vi "updateNots.vi"(8 "error in (no error)":errorcluster, 11 "reference in":refnum<class "Notification Controller.lvclass">) -> (0 "error out":errorcluster, 3 "reference out":refnum<class "Notification Controller.lvclass">)   [LabVIEW 2014, in "Notification Controller.lvclass"]
uses:
  Notification Controller.lvclass
  Devices Controller_llb/deviceType.ctl
  Devices Controller_llb/Devices Controller.lvclass
  APP/itemsNotification_class/itemsNotification.lvclass
  APP/trackingNotification_class/trackingNotification.lvclass
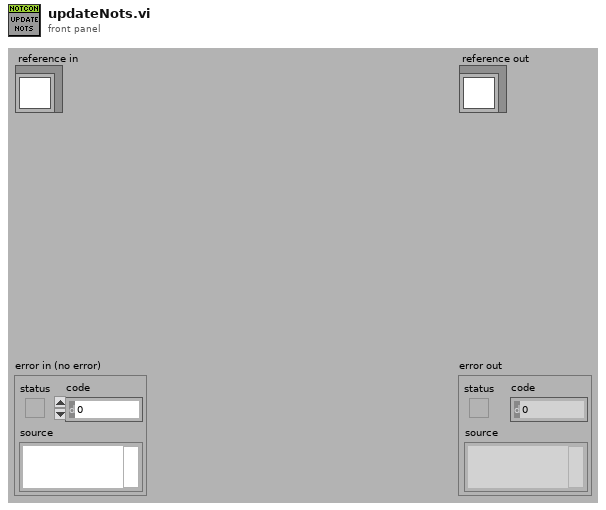
[diagram p1: front panel]
types:
  T1 = typedef "Devices Controller.lvclass/deviceType.ctl" = enum16{"k5", "k4b2", "fitmate", "cpet", "rmr", "bodyBoxPft", "bp", "pp"}
  T2 = cluster{"deviceType":T1, "S/N":string, "SW":string, "Description":string, "Account":string, "System's Location":string, "End User":string, "Email":string, "City":string, "LastChange":string, "Service By":string, "Exp Date":string, "FollowUp Sent":string, "FollowUp Accepted":string, "Note":string}
  T3 = typedef "Notification Controller.lvclass/ObjectAttributesRef.ctl" = refnum<data-value>
  T4 = typedef "Notification Controller.lvclass/ObjectAttributes.ctl" = cluster{"MyAttribute":dbl, "items_data":string[][][], "items_notification_refs":refnum<class "itemsNotification.lvclass">[], "notifications_data_items":string[][], "items_nots?":bool, "devices_controller_ref":refnum<class "Devices Controller.lvclass">, "onlineUpdate":timestamp, "notController?":bool, "tracking_notification_ref":refnum<class "trackingNotification.lvclass">, "notifications_data_tracking":string[][], "tracking_parts_data":string[][], "tracking_nots?":bool, "index_tracking_not":i32[], "file_controller_ref":refnum<class "File Controller.lvclass">}
  T5 = cluster{"notifications_data_items[0]":string, "notifications_data_items[1]":string, "notifications_data_items[2]":string, "notifications_data_items[3]":string, "notifications_data_items[4]":string, "notifications_data_items[5]":string, "notifications_data_items[6]":string, "notifications_data_items[7]":string, "notifications_data_items[8]":string}
  T6 = cluster{"[0]":string, "[1]":string, "[2]":string, "[3]":string, "[4]":string, "[5]":string, "[6]":string, "[7]":string, "[8]":string}
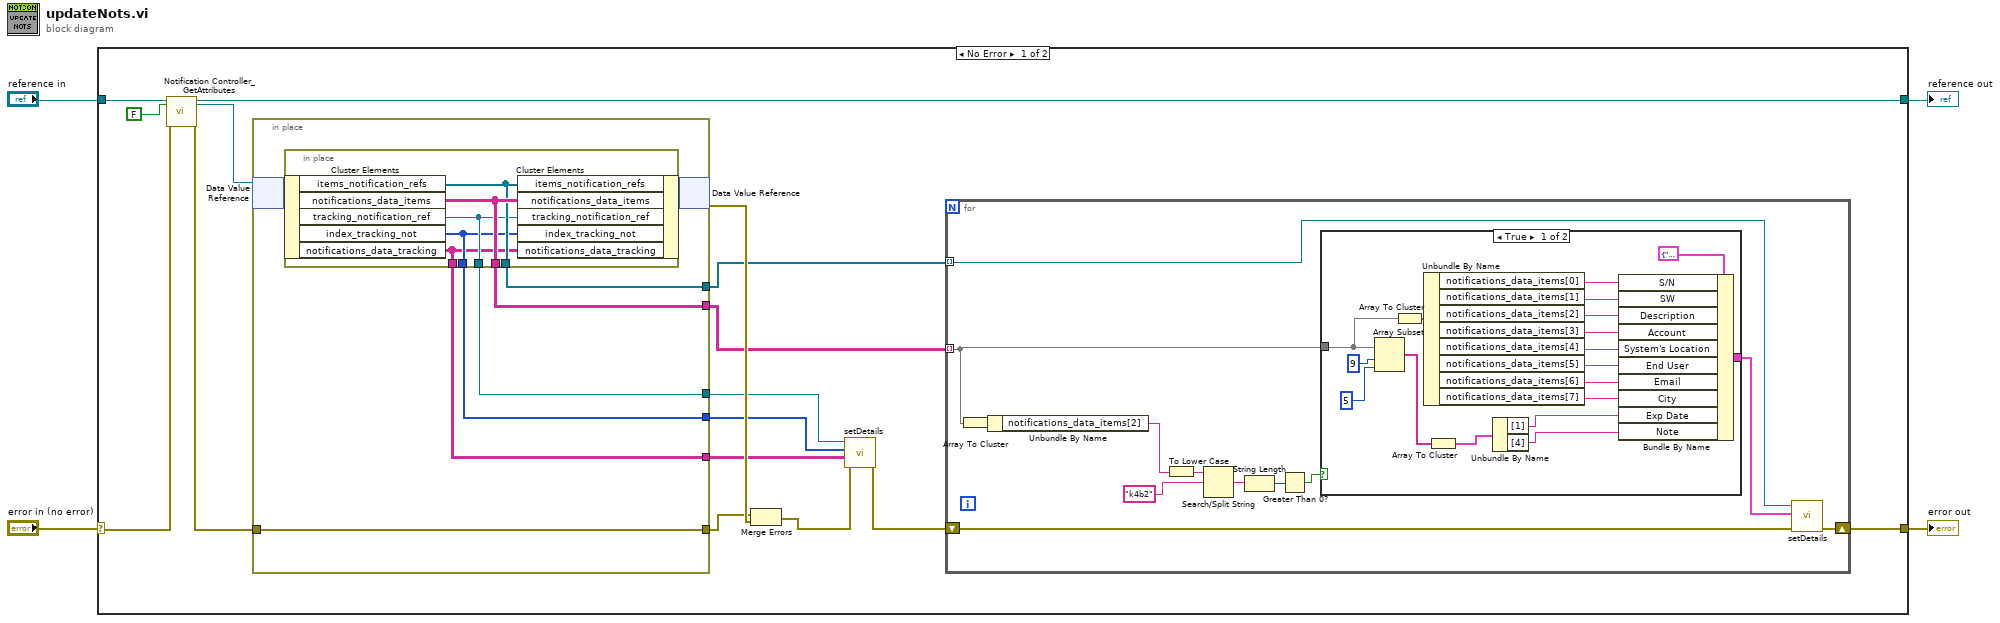
[diagram p0: block diagram]
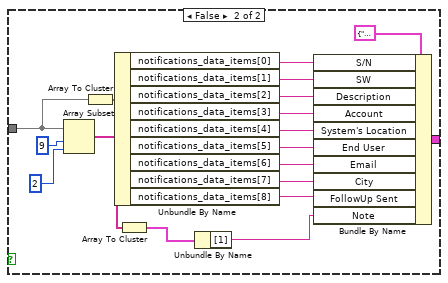
[diagram p2: hidden frame]
diagram:
  n1 = case shown="No Error" "error in (no error)" {
    selector: "error in (no error)" -> [w16 w83]
    tunnel: [w12 w83] -> w3
    tunnel: [w14 w82] -> w1
    tunnel: "reference in" -> [w18 w82]
    frame No Error {
      n2 = call "Notification Controller_GetAttributes.vi"("reference in"=w18, "return data? (T)"=FALSE, "error in (no error)"=w16) -> ("reference out"=w14:refnum<class "Notification Controller.lvclass">, "attributes ref"=w13:T3, "error out"=w15:errorcluster)  [unwired: 13 in, 1 out]
      n3 = in-place {
        in-place-border: w15 -> [w74]
        in-place-border: [w74] -> w19
        in-place-border: [w73] -> w10
        in-place-border: [w72] -> w11
        in-place-border: [w71] -> w9
        in-place-border: [w70] -> w8
        in-place-border: [w69] -> w5
        n4 = in-place-dvr #1(w13) -> (w75:T4)  [unwired: 1 out]
        n5 = in-place {
          in-place-border: [w81] -> w73
          in-place-border: [w80] -> w72
          in-place-border: [w79] -> w71
          in-place-border: [w78] -> w70
          in-place-border: [w77] -> w69
          n6 = in-place-cluster #2(w75) -> ("items_notification_refs"=w80:refnum<class "itemsNotification.lvclass">[], "notifications_data_items"=w81:string[][], "tracking_notification_ref"=w79:refnum<class "trackingNotification.lvclass">, "index_tracking_not"=w78:i32[], "notifications_data_tracking"=w77:string[][])
          n7 = in-place-cluster #2("items_notification_refs"=w80, "notifications_data_items"=w81, "tracking_notification_ref"=w79, "index_tracking_not"=w78, "notifications_data_tracking"=w77) -> (w76:T4)
        }
        n8 = in-place-dvr #1(w76) -> (w20:errorcluster)  [unwired: 1 out]
      }
      n9 = Merge Errors(w19, w20) -> (w7:errorcluster)
      n10 = call "setDetails.vi"("error in (no error)"=w7, "data"=w5, "index_parts_expired"=w8, "reference in"=w9) -> ("error out"=w6:errorcluster)  [unwired: 6 in, 1 out]
      n11 = for {
        tunnel: w11 -> [w30] mode=indexing
        tunnel: w10 -> [w28] mode=indexing
        shift-right: [w31] -> w12
        shift-left: w6 -> [w32]
        n12 = Array To Cluster(array=w28) -> (cluster=w27:T5)
        n13 = Unbundle By Name(w27) -> ("notifications_data_items[2]"=w26:string)
        n14 = To Lower Case(string=w26) -> (all lower case string=w25:string)
        n15 = Search/Split String(string=w25, search string/char (-)="k4b2") -> (match + rest of string=w23:string)  [unwired: 1 in, 2 out]
        n16 = String Length(string=w23) -> (length=w22:i32)
        n17 = Greater Than 0?(x=w22) -> (x > 0?=w21:bool)
        n18 = case shown="True" w21 {
          tunnel: w28 -> [w50 w68]
          tunnel: [w49 w67] -> w29
          frame True {
            n19 = Array Subset(array=w50, index=9, length=5) -> (w45:string[])
            n20 = Array To Cluster(array=w50) -> (cluster=w48:T5)
            n21 = Unbundle By Name(w48) -> ("notifications_data_items[0]"=w43:string, "notifications_data_items[1]"=w42:string, "notifications_data_items[2]"=w41:string, "notifications_data_items[3]"=w40:string, "notifications_data_items[4]"=w39:string, "notifications_data_items[5]"=w38:string, "notifications_data_items[6]"=w37:string, "notifications_data_items[7]"=w36:string)
            n22 = Array To Cluster(array=w45) -> (cluster=w44:T6)
            n23 = Unbundle By Name(w44) -> ("[1]"=w34:string, "[4]"=w33:string)
            n24 = Bundle By Name(cluster=T2 {"deviceType"=enum."k5", "S/N"="", "SW"="", "Description"="", "Account"="", "System's Location"="", "End User"="", "Email"="", "City"="", "LastChange"="", "Service By"="", "Exp Date"="", "FollowUp Sent"="", "FollowUp Accepted"="", "Note"=""} ("details"), "S/N"=w43, "SW"=w42, "Description"=w41, "Account"=w40, "System's Location"=w39, "End User"=w38, "Email"=w37, "City"=w36, "Exp Date"=w34, "Note"=w33) -> (w49:T2)
          }
          frame False {
            n25 = Array Subset(array=w68, index=9, length=2) -> (w63:string[])
            n26 = Array To Cluster(array=w68) -> (cluster=w66:T5)
            n27 = Unbundle By Name(w66) -> ("notifications_data_items[0]"=w61:string, "notifications_data_items[1]"=w60:string, "notifications_data_items[2]"=w59:string, "notifications_data_items[3]"=w58:string, "notifications_data_items[4]"=w57:string, "notifications_data_items[5]"=w56:string, "notifications_data_items[6]"=w55:string, "notifications_data_items[7]"=w54:string, "notifications_data_items[8]"=w51:string)
            n28 = Array To Cluster(array=w63) -> (cluster=w62:T6)
            n29 = Unbundle By Name(w62) -> ("[1]"=w52:string)
            n30 = Bundle By Name(cluster=T2 {"deviceType"=enum."k5", "S/N"="", "SW"="", "Description"="", "Account"="", "System's Location"="", "End User"="", "Email"="", "City"="", "LastChange"="", "Service By"="", "Exp Date"="", "FollowUp Sent"="", "FollowUp Accepted"="", "Note"=""} ("details"), "S/N"=w61, "SW"=w60, "Description"=w59, "Account"=w58, "System's Location"=w57, "End User"=w56, "Email"=w55, "City"=w54, "FollowUp Sent"=w51, "Note"=w52) -> (w67:T2)
          }
        }
        n31 = call "setDetails.vi"("error in (no error)"=w32, "details"=w29, "reference in"=w30) -> ("error out"=w31:errorcluster)  [unwired: 7 in, 1 out]
      }
    }
    frame Error {
    }
  }
  "error out" <- w3
  "reference out" <- w1
